vi "改变光标.vi"(8 "error in (no error)":errorcluster caption="错误输入（无错误）", 11 "程序 输入":refnum<class "程序.lvclass">) -> (0 "error out":errorcluster caption="错误输出", 3 "程序 输出":refnum<class "程序.lvclass">)   [LabVIEW 2018, in "程序.lvclass"]
uses:
  <vilib>/Utility/cursorutil.llb/Set Cursor (Icon Pict).vi
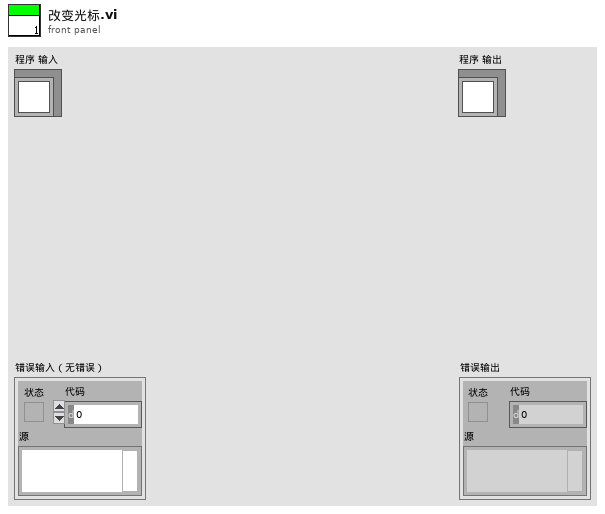
[diagram p1: front panel]
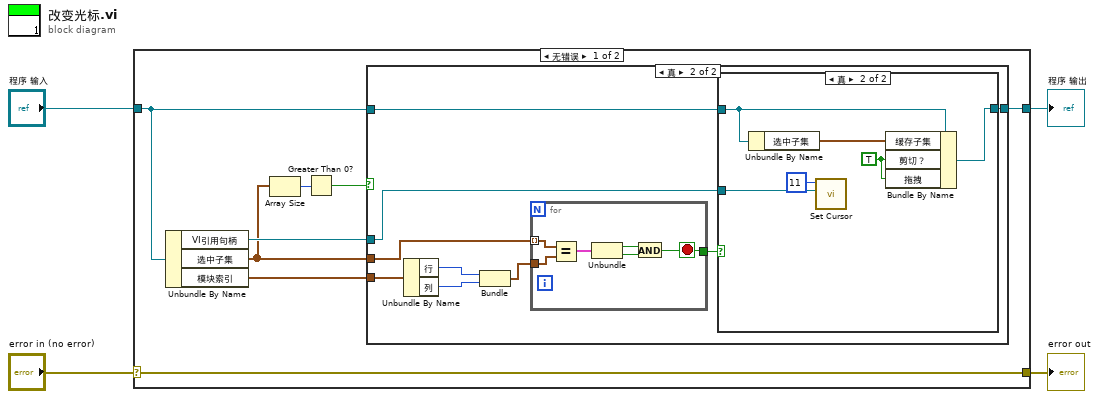
[diagram p0: block diagram]
diagram:
  n1 = case shown="无错误" "error in (no error)" {
    selector: "error in (no error)" -> [w12 w37]
    tunnel: [w12 w37] -> w3
    tunnel: [w8 w36] -> w1
    tunnel: "程序 输入" -> [w9 w36]
    frame No Error {
      n2 = Unbundle By Name(w9) -> ("VI引用句柄"=w10:refnum<vi>, "选中子集"=w5:cluster{"行":i32, "列":i32}[], "模块索引"=w11:cluster{"列":u32, "行":u32})
      n3 = Array Size(array=w5) -> (size(s)=w7:i32)
      n4 = Greater Than 0?(x=w7) -> (x > 0?=w6:bool)
      n5 = case shown="真" w6 {
        tunnel: w11 -> [_ w22]
        tunnel: w5 -> [_ w19]
        tunnel: w10 -> [_ w16]
        tunnel: w9 -> [w13 w15]
        tunnel: [w13 w14] -> w8
        frame False {
        }
        frame True {
          n6 = Unbundle By Name(w22) -> ("行"=w21:u32, "列"=w20:u32)
          n7 = Bundle("行"=w21, "列"=w20) -> (w18:cluster{"行":u32, "列":u32})  [unwired: 1 in]
          n8 = for {
            tunnel: w19 -> [w35] mode=indexing
            tunnel: w18 -> [w34]
            tunnel: [w30] -> w17
            stop <- w30 stop-if-true
            n9 = Equal?(x=w35, y=w34) -> (x = y?=w33:cluster{"行":bool, "列":bool})
            n10 = Unbundle(w33) -> ("行"=w32:bool, "列"=w31:bool)
            n11 = And(x=w32, y=w31) -> (x .and. y?=w30:bool)
          }
          n12 = case shown="真" w17 {
            tunnel: w16 -> [_ w29]
            tunnel: w15 -> [w23 w27]
            tunnel: [w23 w26] -> w14
            frame False {
            }
            frame True {
              w24 = TRUE ("剪切？")
              n13 = Unbundle By Name(w27) -> ("选中子集"=w25:cluster{"行":i32, "列":i32}[])
              n14 = call-poly <vilib>:"Set Cursor.vi"("VI reference (current VI)"=w29, "icon"=u16 11) -> ()  [unwired: 8 in, 2 out]
              n15 = Bundle By Name(cluster=w27, "缓存子集"=w25, "剪切？"=w24, "拖拽"=w24) -> (w26:refnum<class "程序.lvclass">)
            }
          }
        }
      }
    }
    frame Error {
    }
  }
  "error out" <- w3
  "程序 输出" <- w1
